vi "Discard Sub Img Build Bitmap.vi"(9 "Height":i16, 10 "Width":i16, 11 "RGB 8bit Array":u8[](array[numeric])) -> (3 "24-bit pixmap":u32[][](array[numeric]) format="%x")   [LabVIEW 2018]
panel:
  in  "Array":cluster{"R":u8, "G":u8, "B":u8}[](array[cluster])
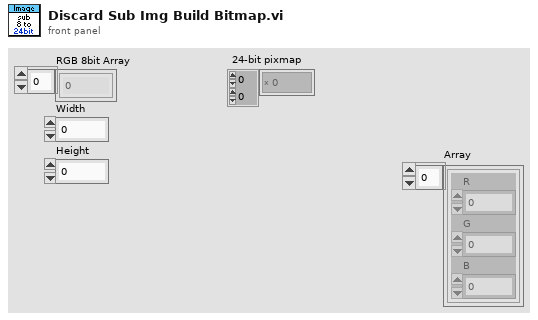
[diagram p1: front panel]
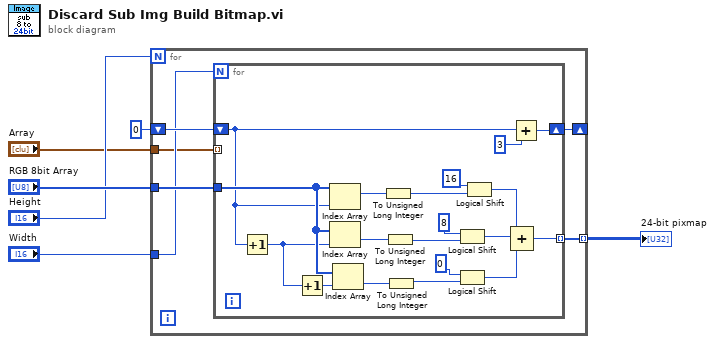
[diagram p0: block diagram]
diagram:
  n1 = for {
    N: "Height" -> [_]
    tunnel: "Width" -> [w8]
    tunnel: "RGB 8bit Array" -> [w12]
    tunnel: [w11] -> w6 mode=indexing
    shift-right: [w9] -> _
    shift-left: 0 -> [w10]
    tunnel: "Array" -> [w7]
    n2 = for {
      N: w8 -> [_]
      tunnel: w12 -> [w31]
      tunnel: [w21] -> w11 mode=indexing
      shift-right: [w19] -> w9
      shift-left: w10 -> [w18]
      tunnel: w7 -> [_] mode=indexing
      n3 = Increment(x=w18) -> (x+1=w17:i32)
      n4 = Increment(x=w17) -> (x+1=w30:i32)
      n5 = Index Array(array=w31, index=w18) -> (element=w24:u8)
      n6 = Index Array(array=w31, index=w17) -> (element=w16:u8)
      n7 = Index Array(array=w31, index=w30) -> (element=w25:u8)
      n8 = To Unsigned Long Integer(number=w24) -> (unsigned 32bit integer=w14:u32)
      n9 = To Unsigned Long Integer(number=w16) -> (unsigned 32bit integer=w27:u32)
      n10 = To Unsigned Long Integer(number=w25) -> (unsigned 32bit integer=w26:u32)
      n11 = Logical Shift(y=i8 8, x=w27) -> (x << y=w23:u32)
      n12 = Logical Shift(y=i8 0, x=w26) -> (x << y=w22:u32)
      n13 = Logical Shift(y=i8 16, x=w14) -> (x << y=w13:u32)
      n14 = Add(x=w18, y=3) -> (x+y=w19:i32)
      n15 = Compound Arithmetic op=ADD(w13, w23, w22) -> (w21:u32)
    }
  }
  "24-bit pixmap" <- w6
